vi "clear Session Data.vi"(0 "OBJ - Measurement Session in":refnum<class "Serial Session.lvclass">, 11 "error in":errorcluster) -> (4 "OBJ - Measurement Session out":refnum<class "Serial Session.lvclass">, 15 "error out":errorcluster)   [LabVIEW 2016, in "Serial Session.lvclass"]
doc: "OVERRIDE VI\nPlaceholder for decendant classes to clear session information and close references."
uses:
  Serial Session.lvclass
  Serial Session.lvclass/Serial Session.ctl
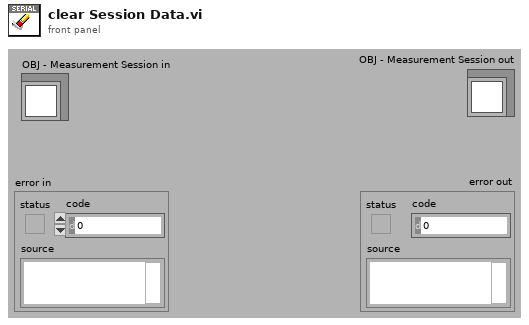
[diagram p1: front panel]
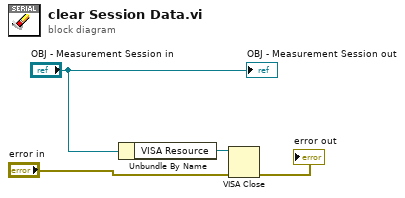
[diagram p0: block diagram]
diagram:
  n1 = Unbundle By Name("OBJ - Measurement Session in") -> ("VISA Resource"=w4:refnum<visa-resource-name>)
  n2 = VISA Close(VISA resource name=w4, error in (no error)="error in") -> (error out=→"error out":errorcluster)
  "OBJ - Measurement Session out" <- "OBJ - Measurement Session in"
